vi "LineStyle.vi"(10 "Line Style":string) -> (2 "Used Line Style":string)   [LabVIEW 2023]
uses:
  <vilib>/Utility/error.llb/whitespace.ctl
  <vilib>/Utility/error.llb/Trim Whitespace One-Sided.vi
panel:
  in  "Default":string="-"
  out "Error":bool
  out "Possible Line Styles":string[](array[string])
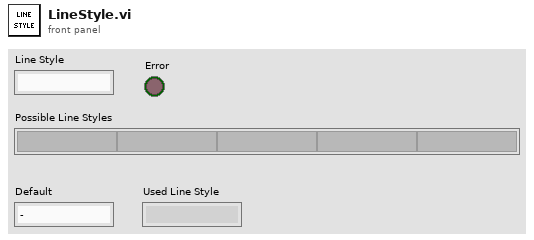
[diagram p1: front panel]
types:
  T1 = typedef "whitespace.ctl" = u16
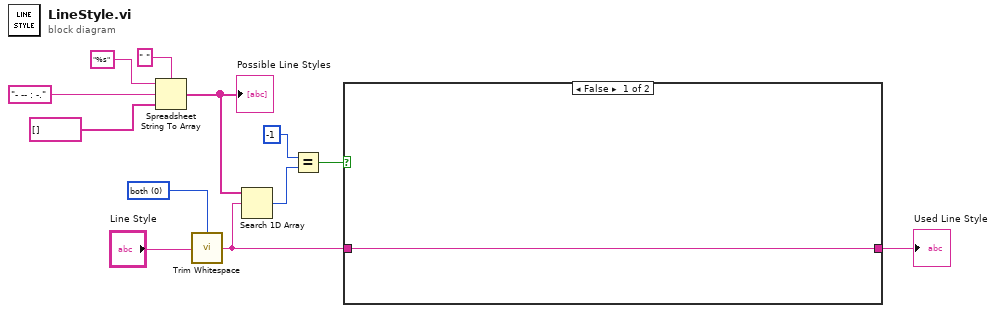
[diagram p0: block diagram]
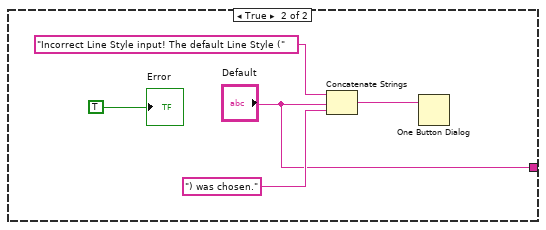
[diagram p2: hidden frame]
diagram:
  w1 = T1 0 items=["both", "start of string", "end of string"] ("location (both)")
  n1 = Spreadsheet String To Array(delimiter (Tab)=" ", format string="%s", spreadsheet string="- -- : -.", array type (2D Dbl)=string[] []) -> (array=w5:string[])
  "Possible Line Styles" <- w5
  n2 = call <vilib>:"Trim Whitespace.vi"("string"="Line Style", "location (both)"=w1) -> ("trimmed string"=w2:string)
  n3 = Search 1D Array(1D array=w5, element=w2) -> (index of element=w10:i32)  [unwired: 1 in]
  n4 = Equal?(x=-1, y=w10) -> (x = y?=w12:bool)
  n5 = case shown="False" w12 {
    tunnel: w2 -> [w13 _]
    tunnel: [w13 "Default"] -> w4
    frame False {
    }
    frame True {
      n6 = Concatenate Strings("Incorrect Line Style input! The default Line Style (", "Default", ") was chosen.") -> (w15:string)
      n7 = One Button Dialog(message=w15) -> ()  [unwired: 1 in, 1 out]
      "Error" <- TRUE
    }
  }
  "Used Line Style" <- w4
